vi "20170516-lecture4-2 queue.vi"() -> ()   [LabVIEW 2014]
panel:
  out "# elements in queue":i32
  out "Tank":dbl(slide) scale=0.0..10.0
  in  "stop":bool
  in  "Wait(ms) in Consumer Loop":u32
  out "Dequeueed Data":string
  in  "Enqueue Data":bool
  in  "Data to Enqueue":string
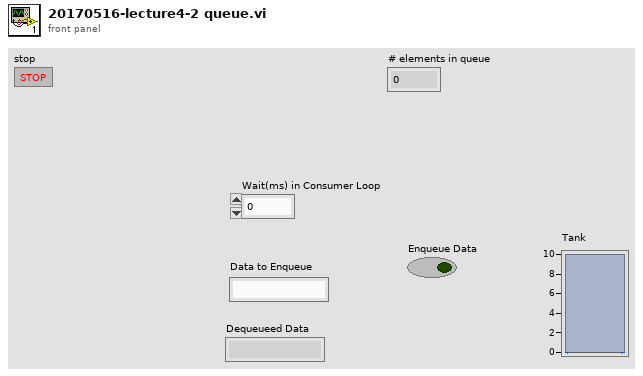
[diagram p1: front panel]
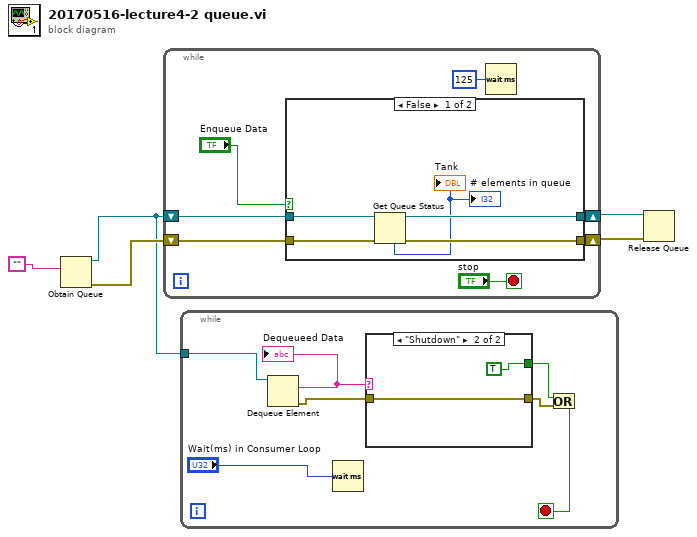
[diagram p0: block diagram]
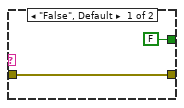
[diagram p2: hidden frame]
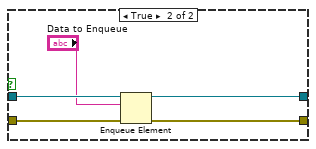
[diagram p3: hidden frame]
diagram:
  n1 = Obtain Queue(element data type="") -> (queue out=w3:refnum<queue>, error out=w4:errorcluster)  [unwired: 4 in, 1 out]
  n2 = while {
    shift-right: [w11] -> w2
    shift-left: w3 -> [w12]
    shift-right: [w9] -> w1
    shift-left: w4 -> [w8]
    stop <- "stop" stop-if-true
    n3 = case shown="False" "Enqueue Data" {
      tunnel: w12 -> [w17 w22]
      tunnel: [w16 w21] -> w11
      tunnel: [w14 w19] -> w9
      tunnel: w8 -> [w15 w18]
      frame False {
        n4 = Get Queue Status(queue=w17, error in (no error)=w15) -> (queue out=w16:refnum<queue>, error out=w14:errorcluster, # elements in queue=→"Tank" →"# elements in queue":i32)  [unwired: 1 in, 5 out]
      }
      frame True {
        n5 = Enqueue Element(queue=w22, element="Data to Enqueue", error in (no error)=w18) -> (queue out=w21:refnum<queue>, error out=w19:errorcluster)  [unwired: 1 in, 1 out]
      }
    }
    n6 = Wait (ms)(milliseconds to wait=u32 125) -> ()  [unwired: 1 out]
  }
  n7 = while {
    tunnel: w3 -> [w29]
    stop <- w26 stop-if-true
    n8 = Dequeue Element(queue=w29) -> (element=w28:string, error out=w25:errorcluster)  [unwired: 2 in, 2 out]
    "Dequeueed Data" <- w28
    n9 = Wait (ms)(milliseconds to wait="Wait(ms) in Consumer Loop") -> ()  [unwired: 1 out]
    n10 = case shown="\"Shutdown\"" w28 {
      tunnel: [w31 w33] -> w23
      tunnel: w25 -> [w31 w33]
      tunnel: [FALSE ("x .or. y?") TRUE ("x .or. y?")] -> w24
      frame "False", Default {
      }
      frame "Shutdown" {
      }
    }
    n11 = Or(x=w24, y=w23) -> (x .or. y?=w26:bool)
  }
  n12 = Release Queue(queue=w2, error in (no error)=w1) -> ()  [unwired: 1 in, 3 out]
